vi "WASH error handler.vi"(7 "task":T1=enum."handle error", 8 "error in (no error)":errorcluster, 10 "step name":string, 11 "error levels":T2) -> (0 "error out":errorcluster, 1 "system error?":bool, 2 "wash cycle error?":bool)   [LabVIEW 2012]
doc: "handles application errors."
uses:
  type defs/WASH error levels.ctl
  type defs/WASh error handler tasks.ctl
panel:
  in  "station name":string
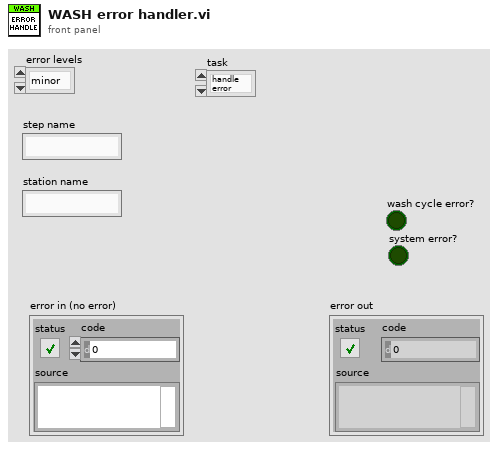
[diagram p1: front panel]
types:
  T1 = typedef "WASh error handler tasks.ctl" = enum16{"init", "set current step", "handle error", "close"}
  T2 = typedef "WASH error levels.ctl" = enum16{"minor", "wash cycle", "system"}
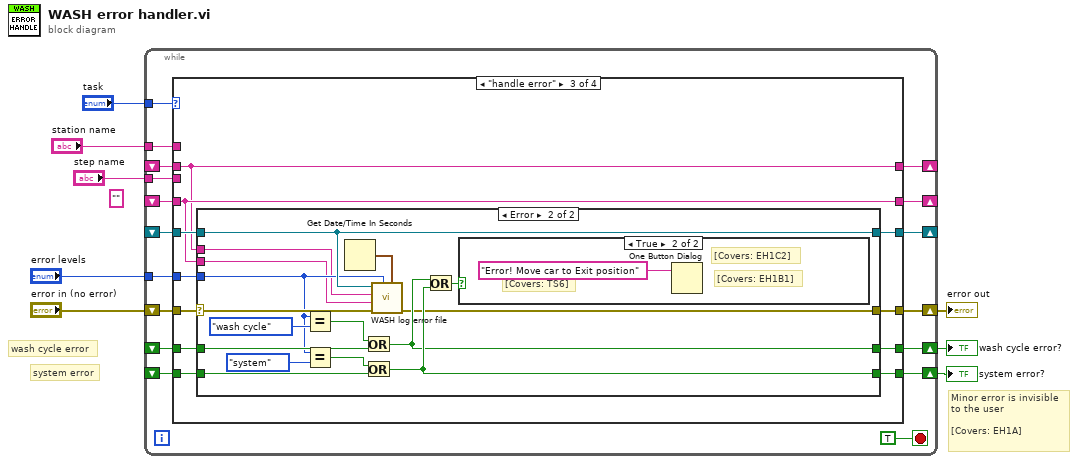
[diagram p0: block diagram]
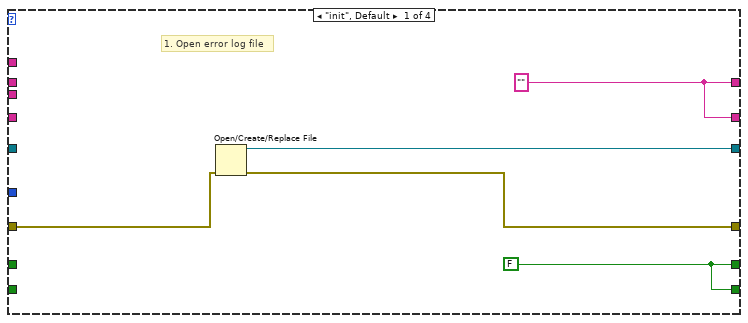
[diagram p2: hidden frame]
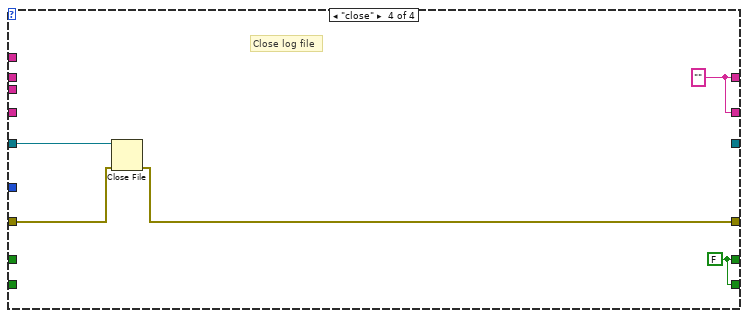
[diagram p6: hidden frame]
diagram:
  (unwired) "" ("step name")
  # "Minor error is invisible\nto the user\n\n[Covers: EH1A]"
  # "system error"
  # "wash cycle error"
  n1 = while {
    tunnel: "task" -> [w24]
    shift-right: [w23] -> _
    shift-left: _ -> [w20]
    shift-right: [w19] -> w6
    shift-left: _ -> [w13]
    shift-right: [w18] -> w5
    shift-left: _ -> [w12]
    shift-right: [w22] -> _
    shift-left: _ -> [w17]
    tunnel: "step name" -> [w21]
    shift-right: [w15] -> w3
    shift-left: "error in (no error)" -> [w16]
    tunnel: "error levels" -> [w14]
    shift-right: [w11] -> _
    shift-left: _ -> [w9]
    tunnel: "station name" -> [w10]
    stop <- TRUE stop-if-true
    n2 = case shown="\"handle error\"" w24 {
      tunnel: [w30 w35 w44 _] -> w23
      tunnel: [w28 w36 w38 w73] -> w22
      tunnel: w21 -> [_ w36 _ _]
      tunnel: w20 -> [_ w35 w45 w71]
      tunnel: [w29 w34 w41 w72] -> w19
      tunnel: [w29 w33 w39 w72] -> w18
      tunnel: w17 -> [_ _ w38 _]
      tunnel: w16 -> [w26 w32 w47 w70]
      tunnel: [w27 w32 w46 w69] -> w15
      tunnel: w14 -> [_ _ w43 _]
      tunnel: w13 -> [_ w34 w42 _]
      tunnel: w12 -> [_ w33 w40 _]
      tunnel: [w28 w31 w37 w73] -> w11
      tunnel: w10 -> [_ w31 _ _]
      tunnel: w9 -> [_ _ w37 _]
      frame "init", Default {
        w29 = FALSE
        w28 = "" ("step name")
        # "1. Open error log file"
        n3 = Open/Create/Replace File(error in=w26) -> (refnum out=w30:refnum<file>, error out=w27:errorcluster)  [unwired: 5 in, 1 out]
      }
      frame "set current step" {
      }
      frame "handle error" {
        n4 = case shown="Error" w47 {
          selector: w47 -> [w51 w58]
          tunnel: [w51 w57] -> w46
          tunnel: w45 -> [w50 w56]
          tunnel: [w50 w56] -> w44
          tunnel: w43 -> [_ w55]
          tunnel: w42 -> [w49 w64]
          tunnel: [w49 w60] -> w41
          tunnel: w40 -> [w48 w63]
          tunnel: [w48 w61] -> w39
          tunnel: w38 -> [_ w53]
          tunnel: w37 -> [_ w54]
          frame No Error {
            # "Continue operating"
          }
          frame Error {
            n5 = Equal?(x=w55, y=WASH_error_levels."wash cycle") -> (x = y?=w65:bool)
            n6 = Equal?(x=w55, y=WASH_error_levels."system") -> (x = y?=w62:bool)
            n7 = Get Date/Time In Seconds() -> (seconds since 1Jan1904=w52:timestamp)
            n8 = Or(x=w65, y=w64) -> (x .or. y?=w60:bool)
            n9 = Or(x=w62, y=w63) -> (x .or. y?=w61:bool)
            n10 = call "WASH log error file.vi"("Time Stamp"=w52, "error levels"=w55, "error in (no error)"=w58, "step name"=w53, "station name"=w54, "refnum out"=w56) -> ("error out"=w57:errorcluster)  [unwired: 5 in]
            n11 = Or(x=w60, y=w61) -> (x .or. y?=w59:bool)
            n12 = case shown="True" w59 {
              frame False {
              }
              frame True {
                # "[Covers: TS6]"
                # "[Covers: EH1C2]"
                # "[Covers: EH1B1]"
                n13 = One Button Dialog(message="Error! Move car to Exit position") -> ()  [unwired: 1 in, 1 out]
              }
            }
          }
        }
      }
      frame "close" {
        w72 = FALSE
        w73 = "" ("station name")
        # "Close log file"
        n14 = Close File(refnum=w71, error in=w70) -> (error out=w69:errorcluster)  [unwired: 1 out]
      }
    }
  }
  "wash cycle error?" <- w6
  "system error?" <- w5
  "error out" <- w3
